vi "DriveBrake.vi"(1 "Butterfly State In":bool=TRUE) -> (0 "Butterfly State Out":bool)   [LabVIEW 2018]
uses:
  Inputs_DriverStation.vi
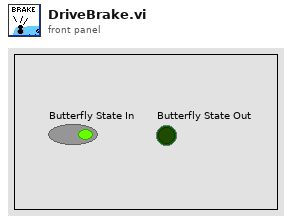
[diagram p1: front panel]
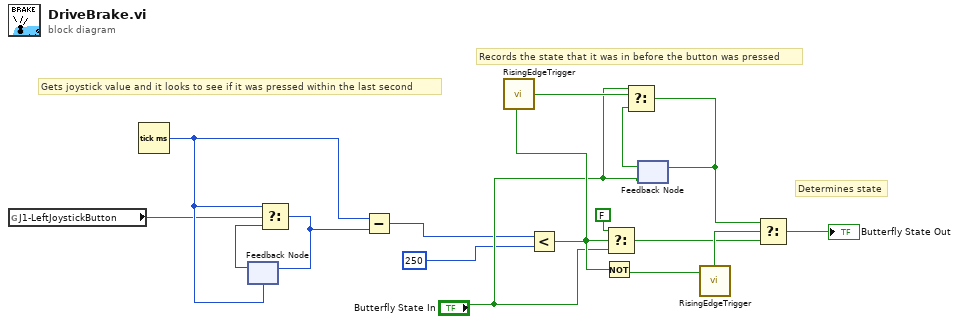
[diagram p0: block diagram]
diagram:
  # "Determines state"
  # "Records the state that it was in before the button was pressed"
  # "Gets joystick value and it looks to see if it was pressed within the last second"
  n1 = global read "Inputs_DriverStation.vi" "J1-LeftJoystickButton"() -> (w3:bool)
  n2 = Tick Count (ms)() -> (millisecond timer value=w4:u32)
  n3 = feedback #1(w4) -> (w2:u32)
  n4 = Select(t=w4, s=w3, f=w2) -> (s? t:f=w5:u32)
  n5 = feedback-in #1(w5) -> ()
  n6 = Subtract(x=w4, y=w5) -> (x-y=w6:u32)
  n7 = Less?(x=w6, y=u32 250) -> (x < y?=w15:bool)
  n8 = call "RisingEdgeTrigger.vi"("Raw Signal"=w15) -> ("Trigger"=w16:bool)
  n9 = Not(x=w15) -> (.not. x?=w10:bool)
  n10 = Select(t=FALSE, s=w15, f="Butterfly State In") -> (s? t:f=w9:bool)
  n11 = feedback #2("Butterfly State In") -> (w13:bool)
  n12 = Select(t="Butterfly State In", s=w16, f=w13) -> (s? t:f=w12:bool)
  n13 = feedback-in #2(w12) -> ()
  n14 = call "RisingEdgeTrigger.vi"("Raw Signal"=w10) -> ("Trigger"=w11:bool)
  n15 = Select(t=w12, s=w11, f=w9) -> (s? t:f=→"Butterfly State Out":bool)
